vi "array.vi"() -> ()   [LabVIEW 2025]
panel:
  out "arr":dbl[](array[numeric])
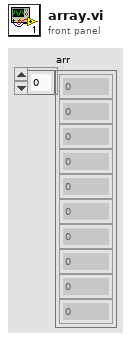
[diagram p1: front panel]
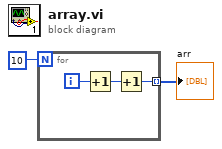
[diagram p0: block diagram]
diagram:
  n1 = for {
    N: 10 -> [_]
    tunnel: [w3] -> w1 mode=indexing
    i -> [w5]
    n2 = Increment(x=w5) -> (x+1=w4:i32)
    n3 = Increment(x=w4) -> (x+1=w3:i32)
  }
  "arr" <- w1
